vi "Save to File.vi"(8 "error in (no error)":errorcluster, 10 "digital audio protocol settings":T1={"number of channels"=0, "data justification"=enum."Left Justified", "endianness"=enum."LSB First", "channel length"=0, "bit depth"=0, "frame clock rate"=0.0, "bit clock edge sync"=enum."Falling", "master clock rate"=0.0, "Logic Level"=enum."1.2 V", "frame sync edge for channel 0"=enum."Rising", "Channel 0 Offset"=0}, 11 "file path":path) -> (0 "error out":errorcluster)   [LabVIEW 2021, in "digital audio protocol controls.lvlib"]
uses:
  digital audio protocol controls.lvlib
  digital audio protocol settings.ctl
  <vilib>/PDM Acquisition Toolkit/shared/controls/PCM Data Justification.ctl
  <vilib>/PDM Acquisition Toolkit/shared/controls/PCM Bit Endianness.ctl
  <vilib>/PDM Acquisition Toolkit/shared/controls/Digital Edge.ctl
  <vilib>/PDM Acquisition Toolkit/host/Classes/Session/Controls/Logic Levels.ctl
  <vilib>/PDM Acquisition Toolkit/shared/PDM Shared.lvlib
  <vilib>/PDM Acquisition Toolkit/host/Classes/Session/DecoderSession.lvclass
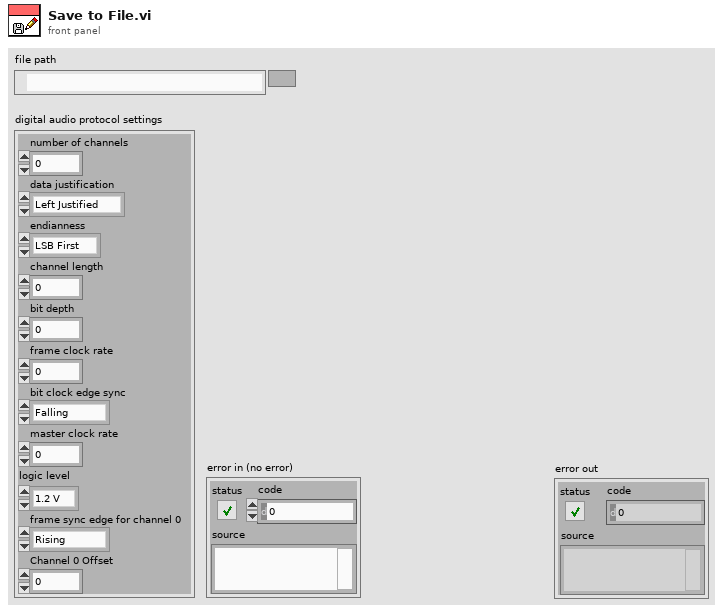
[diagram p1: front panel]
types:
  T1 = typedef "digital audio protocol controls.lvlib/digital audio protocol settings.ctl" = cluster{"number of channels":u32, "data justification":T2, "endianness":T3, "channel length":u32, "bit depth":u32, "frame clock rate":dbl, "bit clock edge sync":T4, "master clock rate":dbl, "Logic Level":T5, "frame sync edge for channel 0":T4, "Channel 0 Offset":u32}
  T2 = typedef "PDM Shared.lvlib/PCM Data Justification.ctl" = enum16{"Left Justified", "Right Justified"}
  T3 = typedef "PDM Shared.lvlib/PCM Bit Endianness.ctl" = enum16{"MSB First", "LSB First"}
  T4 = typedef "PDM Shared.lvlib/Digital Edge.ctl" = enum8{"Rising", "Falling"}
  T5 = typedef "PDM Acquisition Class Library.lvlib/DecoderSession.lvclass/Logic Levels.ctl" = enum16{"3.3 V", "1.8 V", "1.2 V"}
  T6 = typedef "digital audio protocol controls.lvlib/digital audio protocol settings_json.ctl" = cluster{"number of channels":u32, "data justification":string, "endianness":string, "channel length":u32, "bit depth":u32, "frame clock rate":dbl, "bit clock edge sync":string, "master clock rate":dbl, "logic level":string, "frame sync edge for channel 0":string, "Channel 0 Offset":u32}
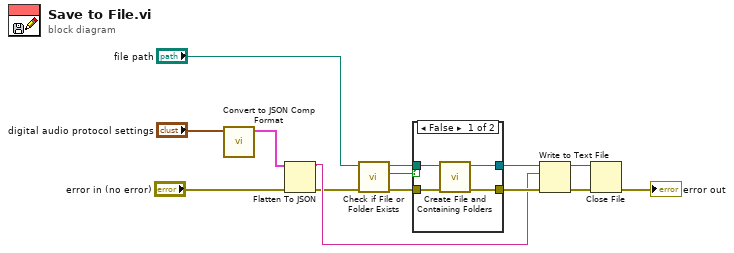
[diagram p0: block diagram]
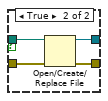
[diagram p2: hidden frame]
diagram:
  n1 = call "Convert to JSON Comp Format.vi"("digital audio protocol settings"="digital audio protocol settings") -> ("JSON compatible settings"=w12:T6)  [unwired: 10 in]
  n2 = Flatten To JSON(anything=w12, error in (no error)="error in (no error)") -> (JSON string=w6:string, 11:w5:errorcluster)  [unwired: 1 in]
  n3 = call <vilib>:"Check if File or Folder Exists.vi"("error in (no error)"=w5, "path"="file path") -> ("error out"=w3:errorcluster, "file or folder exists?"=w2:bool, "dup path"=w1:path)  [unwired: 7 in]
  n4 = case shown="False" w2 {
    tunnel: [w18 w22] -> w11
    tunnel: [w17 w19] -> w10
    tunnel: w3 -> [w16 w20]
    tunnel: w1 -> [w15 w21]
    frame False {
      n5 = call <vilib>:"Create File and Containing Folders.vi"("error in (no error)"=w16, "file path"=w15) -> ("error out"=w18:errorcluster, "refnum out"=w17:refnum<file>)  [unwired: 8 in]
    }
    frame True {
      n6 = Open/Create/Replace File(file path (use dialog)=w21, error in=w20) -> (refnum out=w19:refnum<file>, error out=w22:errorcluster)  [unwired: 4 in, 1 out]
    }
  }
  n7 = Write to Text File(file (use dialog)=w10, text=w6, error in=w11) -> (refnum out=w8:refnum<file>, error out=w9:errorcluster)  [unwired: 1 in, 1 out]
  n8 = Close File(refnum=w8, error in=w9) -> (error out=→"error out":errorcluster)  [unwired: 1 out]
